vi "Test Speed Of Norwegian Blue Parrot Not Nailed.vi"(8 "error in":errorcluster, 11 "Test Parrot in":refnum<class "Test Parrot.lvclass">) -> (0 "error out":errorcluster, 3 "Test Parrot out":refnum<class "Test Parrot.lvclass">)   [LabVIEW 2020, in "Test Parrot.lvclass"]
uses:
  Test Parrot.lvclass
  C:/Program Files/National Instruments/LabVIEW 2025/vi.lib/Astemes/LUnit/Test Case.lvclass
  <vilib>/Astemes/LUnit/Test Case.lvclass/Test Case.ctl
  Parrot/Parrot.lvclass
  5cc24d4d-52ce-4497-bd59-7a92c8fac89d.vi
  Parrot/Parrot Type.ctl
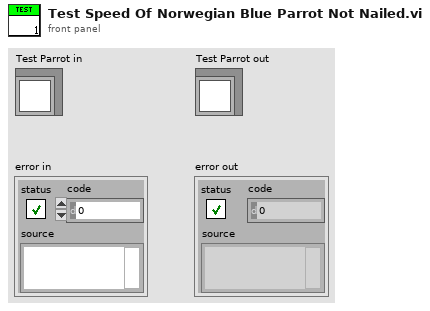
[diagram p1: front panel]
types:
  T1 = typedef "Parrot.lvclass/Parrot Type.ctl" = enum16{"European", "African", "Norwegian Blue"}
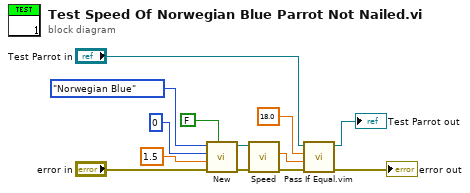
[diagram p0: block diagram]
diagram:
  n1 = call "New.vi"("Nailed?"=FALSE, "error in"="error in", "Voltage"=1.5, "Number of Coconuts"=0, "Type of Parrot"=Parrot_Type."Norwegian Blue") -> ("error out"=w12:errorcluster, "Parrot out"=w9:refnum<class "Parrot.lvclass">)  [unwired: 5 in]
  n2 = call-dynamic "Speed.vi"("error in"=w12, "Parrot in"=w9) -> ("error out"=w11:errorcluster, "Speed"=w6:dbl)  [unwired: 7 in, 1 out]
  n3 = call "Pass If Equal.vim"("error in (no error)"=w11, "Actual"=w6, "Expected"=18.0, "LUnit Test Case In"="Test Parrot in") -> ("error out"=→"error out":errorcluster, "LUnit Test Case Out"=→"Test Parrot out":refnum<class "Test Parrot.lvclass">)  [unwired: 6 in]
